vi "mcc_usb202_test.vi"(6 "error in":errorcluster) -> (4 "error out":errorcluster={"status"=TRUE, "code"=10023, "source"="ULx Create Channel (AI-Voltage-Basic).vi:5780001<ERR>\nMeasurements: Channel not specified."})   [LabVIEW 2019]
panel:
  out "V1":dbl
  out "V0":dbl
  out "i":i32
  in  "stop":bool
  out "Time":timestamp format="%<%Y-%m-%d %H:%M:%S>T"
  out "status_close":bool=TRUE
  out "status_read":bool=TRUE
  out "status_open":bool=TRUE
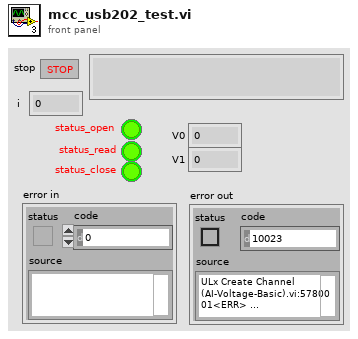
[diagram p1: front panel]
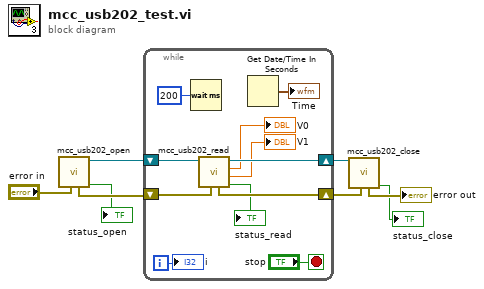
[diagram p0: block diagram]
diagram:
  n1 = call "mcc_usb202_open.vi"("error in"="error in") -> ("status"=→"status_open":bool, "task out"=w7:refnum<k24>, "error out"=w6:errorcluster)  [unwired: 8 in]
  n2 = while {
    shift-right: [w17] -> w5
    shift-left: w7 -> [w19]
    shift-right: [w16] -> w4
    shift-left: w6 -> [w18]
    i -> [w12]
    stop <- "stop" stop-if-true
    n3 = Wait (ms)(milliseconds to wait=u32 200) -> ()  [unwired: 1 out]
    n4 = call "mcc_usb202_read.vi"("error in"=w18, "task in"=w19) -> ("status"=→"status_read":bool, "V1"=→"V1":dbl, "V0"=→"V0":dbl, "task out"=w17:refnum<k24>, "error out"=w16:errorcluster)  [unwired: 5 in]
    n5 = Get Date/Time In Seconds() -> (seconds since 1Jan1904=→"Time":timestamp)
    "i" <- w12
  }
  n6 = call "mcc_usb202_close.vi"("error in"=w4, "task in"=w5) -> ("status"=→"status_close":bool, "error out"=→"error out":errorcluster)  [unwired: 8 in]
